vi "Serialize CVT.vi"(11 "force?":bool) -> (0 "error out":errorcluster, 3 "json out":string)   [LabVIEW 2017, in "Controller.lvlib" / "gController.lvclass"]
uses:
  gController.lvclass
  <vilib>/MSR Consulting, LLC/General Reuse/Session APIs/CVT/CVT.lvclass
  C:/Program Files (x86)/National Instruments/LabVIEW 2017/vi.lib/MSR Consulting, LLC/General Reuse/Session APIs/_Session Fwk/Session - Root.lvclass
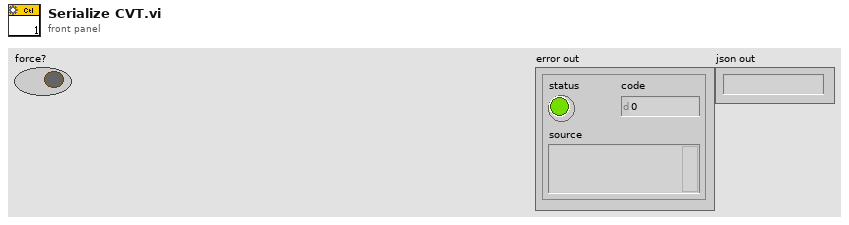
[diagram p1: front panel]
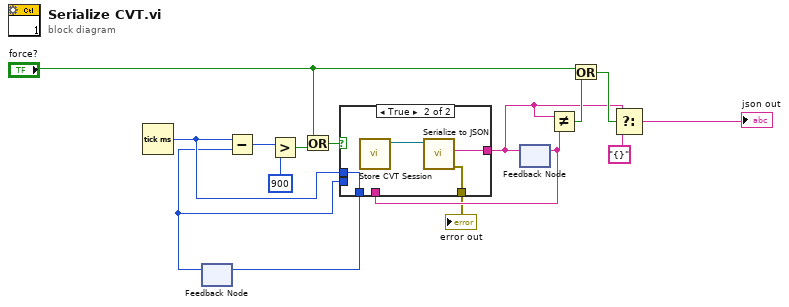
[diagram p0: block diagram]
diagram:
  n1 = Tick Count (ms)() -> (millisecond timer value=w9:u32)
  n2 = feedback #1() -> (w7:u32)  [unwired: 1 in]
  n3 = Subtract(x=w9, y=w7) -> (x-y=w12:u32)
  n4 = Greater?(x=w12, y=u32 900) -> (0:w10:bool)
  n5 = Or(x="force?", y=w10) -> (x .or. y?=w1:bool)
  n6 = feedback #2() -> (w6:string)  [unwired: 1 in]
  n7 = case shown="True" w1 {
    tunnel: [_ w20] -> w3
    tunnel: [w17 w19] -> w5
    tunnel: w6 -> [w17 _]
    tunnel: w9 -> [_ w18]
    tunnel: [w16 w18] -> w8
    tunnel: w7 -> [w16 _]
    frame False {
    }
    frame True {
      n8 = call "Store CVT Session.vi"() -> ("CVT Session Out"=w21:refnum<data-value>)  [unwired: 11 in]
      n9 = call <vilib>:"Serialize to JSON.vi"("CVT Session In"=w21) -> ("error out"=w20:errorcluster, "SerializedString"=w19:string)  [unwired: 8 in, 1 out]
    }
  }
  "error out" <- w3
  n10 = feedback-in #1(w8) -> ()
  n11 = feedback-in #2(w5) -> ()
  n12 = Not Equal?(x=w5, y=w6) -> (x != y?=w14:bool)
  n13 = Or(x="force?", y=w14) -> (x .or. y?=w15:bool)
  n14 = Select(t=w5, s=w15, f="{}") -> (s? t:f=→"json out":string)
